vi "Magnetic Field Lakeshore Scan.vi"(8 "error in (no error)":errorcluster, 10 "Lakeshore Gaussmeter.lvclass":refnum<class "Lakeshore Gaussmeter.lvclass">, 11 "Magnetic Field Lakeshore Scan in":refnum<class "Magnetic Field Lakeshore Scan.lvclass">) -> (0 "error out":errorcluster, 3 "Magnetic Field Lakeshore Scan out":refnum<class "Magnetic Field Lakeshore Scan.lvclass">)   [LabVIEW 2017, in "Magnetic Field Lakeshore Scan.lvclass"]
uses:
  Magnetic Field Lakeshore Scan.lvclass
  C:/LabVIEW-programs/Scanners/Scanner/Scanner.lvclass
  Instruments/Lakeshore Gaussmeter/Lakeshore Gaussmeter.lvclass
  C:/LabVIEW-programs/Instruments/Utility Classes/Scannable/Scannable.lvclass
  Scanner/Scanner.lvclass
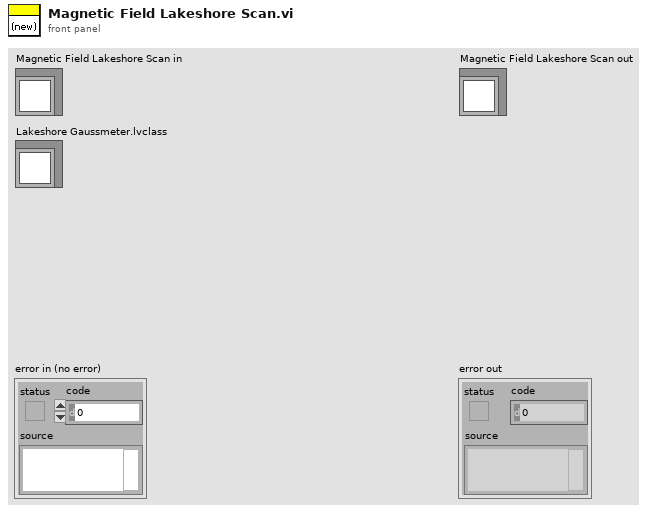
[diagram p1: front panel]
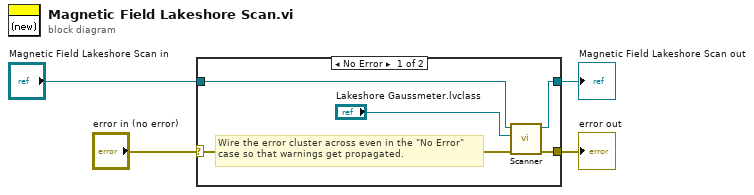
[diagram p0: block diagram]
diagram:
  n1 = case shown="No Error" "error in (no error)" {
    selector: "error in (no error)" -> [w6 w11]
    tunnel: [w5 w11] -> w3
    tunnel: [w7 w10] -> w1
    tunnel: "Magnetic Field Lakeshore Scan in" -> [w8 w10]
    frame No Error {
      # "Wire the error cluster across even in the \"No Error\"\ncase so that warnings get propagated."
      n2 = call "Scanner.vi"("error in (no error)"=w6, "Scannable"="Lakeshore Gaussmeter.lvclass", "Scanner.lvclass in"=w8) -> ("error out"=w5:errorcluster, "Scanner.lvclass out"=w7:refnum<class "Magnetic Field Lakeshore Scan.lvclass">)  [unwired: 1 in, 6 out]
    }
    frame Error {
    }
  }
  "error out" <- w3
  "Magnetic Field Lakeshore Scan out" <- w1
